vi "SUB_s8300E-TestPoint_Format.vi"(0 "TestPoint_Name":string="TP46", 1 "Lower Limit Voltage":dbl format="%#.6f", 3 "High Limit Voltage":dbl format="%#.6f", 4 "Relay 1 Name":string, 5 "Relay1 H/L":bool=TRUE, 8 "Relay 2 Name":string, 9 "Relay2 H/L":bool=TRUE, 12 "Relay3 Name":string, 13 "Relay3H/L":bool=TRUE, 14 "Measure Ai name":string, 16 "Relay4 Name":string, 17 "Relay4 H/L":bool=TRUE, 18 "Relay5 Name":string, 19 "Relay5 H/L":bool=TRUE) -> (20 "output cluster":T1 {"Lower Limit Voltage" format="%#.6f"; "High Limit Voltage" format="%#.6f"})   [LabVIEW 2011]
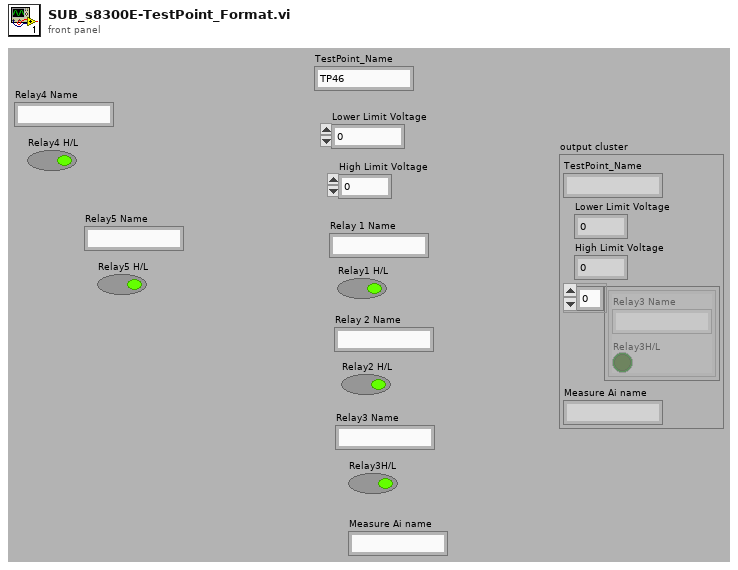
[diagram p1: front panel]
types:
  T1 = cluster{"TestPoint_Name":string, "Lower Limit Voltage":dbl, "High Limit Voltage":dbl, cluster{"Relay3 Name":string, "Relay3H/L":bool}[], "Measure Ai name":string}
  T2 = cluster{"Relay 1 Name":string, "Relay1 H/L":bool}
  T3 = cluster{"Relay 2 Name":string, "Relay2 H/L":bool}
  T4 = cluster{"Relay4 Name":string, "Relay4 H/L ":bool}
  T5 = cluster{"Relay5 Name":string, "Relay5 H/L":bool}[]
  T6 = cluster{"TestPoint_Name":string, "Lower Limit Voltage":dbl, "High Limit Voltage ":dbl, cluster{"Relay5 Name":string, "Relay5 H/L":bool}[], "Measure Ai name":string}
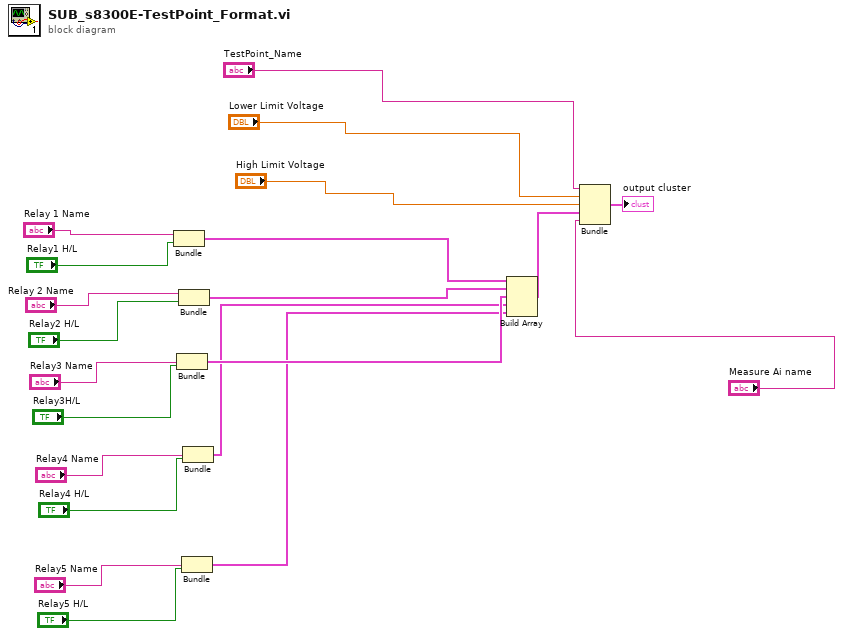
[diagram p0: block diagram]
diagram:
  n1 = Bundle("Relay 1 Name"="Relay 1 Name", "Relay1 H/L"="Relay1 H/L") -> (w15:T2)  [unwired: 1 in]
  n2 = Bundle("Relay3 Name"="Relay3 Name", "Relay3H/L"="Relay3H/L") -> (w13:cluster{"Relay3 Name":string, "Relay3H/L":bool})  [unwired: 1 in]
  n3 = Bundle("Relay 2 Name"="Relay 2 Name", "Relay2 H/L"="Relay2 H/L") -> (w14:T3)  [unwired: 1 in]
  n4 = Bundle("Relay5 Name"="Relay5 Name", "Relay5 H/L"="Relay5 H/L") -> (w1:cluster{"Relay5 Name":string, "Relay5 H/L":bool})  [unwired: 1 in]
  n5 = Bundle("Relay4 Name"="Relay4 Name", "Relay4 H/L"="Relay4 H/L") -> (w2:T4)  [unwired: 1 in]
  n6 = Build Array(w15, w14, w13, w2, w1) -> (w9:T5)
  n7 = Bundle("TestPoint_Name"="TestPoint_Name", "Lower Limit Voltage"="Lower Limit Voltage", "High Limit Voltage"="High Limit Voltage", w9, "Measure Ai name"="Measure Ai name") -> (→"output cluster":T6)  [unwired: 1 in]
